vi "create Disconnect.vi"(8 "error in (no error)":errorcluster, 10 "Player":refnum<class "Player.lvclass">, 11 "Disconnect in":refnum<class "Disconnect.lvclass">) -> (0 "error out":errorcluster, 3 "Disconnect out":refnum<class "Disconnect.lvclass">)   [LabVIEW 2019, in "Disconnect.lvclass"]
uses:
  Disconnect.lvclass
  Player/Player.lvclass
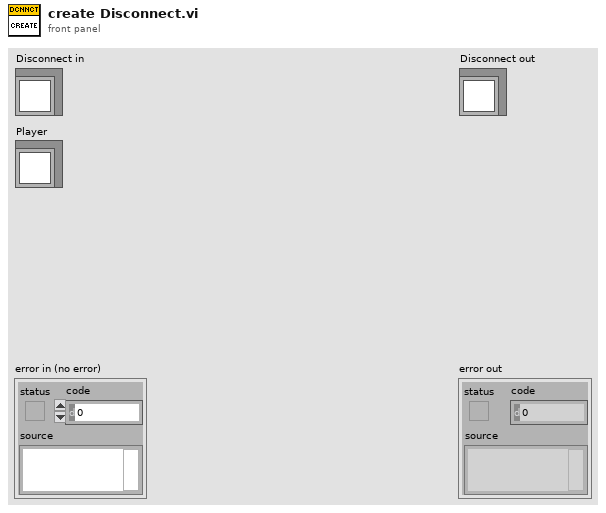
[diagram p1: front panel]
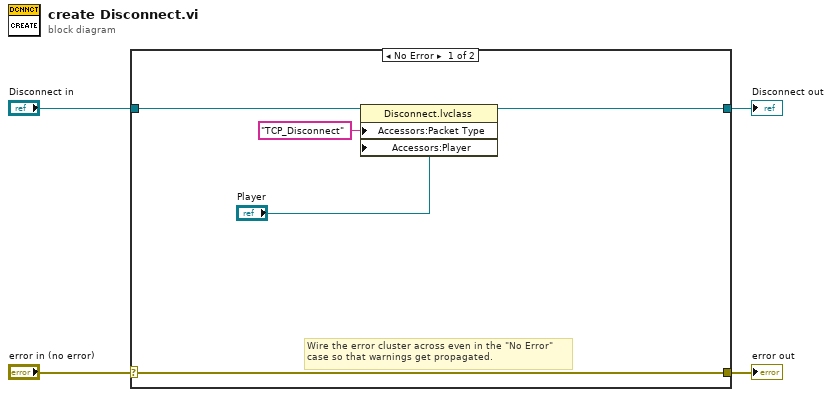
[diagram p0: block diagram]
diagram:
  n1 = case shown="No Error" "error in (no error)" {
    selector: "error in (no error)" -> [w9 w11]
    tunnel: [w9 w11] -> w3
    tunnel: [w7 w10] -> w1
    tunnel: "Disconnect in" -> [w8 w10]
    frame No Error {
      # "Wire the error cluster across even in the \"No Error\"\ncase so that warnings get propagated."
      n2 = property class="Disconnect.lvclass"(reference=w8, "Accessors:Packet Type"="TCP_Disconnect" ("Packet Type"), "Accessors:Player"="Player") -> (reference out=w7:refnum<class "Disconnect.lvclass">)  [unwired: 1 in, 1 out]
    }
    frame Error {
    }
  }
  "error out" <- w3
  "Disconnect out" <- w1
